vi "PH_SRDG645.calc Device Errors.vi"(1 "Device Errors out":cluster{"code":i32, "Text":string}[](array[cluster]), 2 "SRDG 645 error out":errorcluster) -> (0 "calculate Device Errors":cluster{"code":i32, "Text":string}[](array[cluster]))   [LabVIEW 2014, in "PH_SRDG645.lvlib"]
doc: "This VI calöculates the Device Errors; if \"Device Errors out\" are empty, \"SRDG 645 Error out\" is taken."
uses:
  PH_SRDG645.lvlib
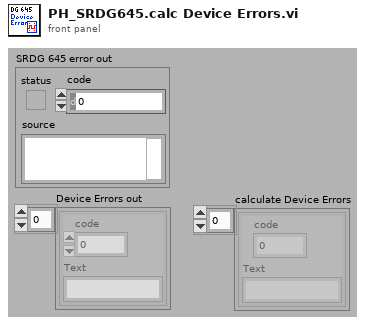
[diagram p1: front panel]
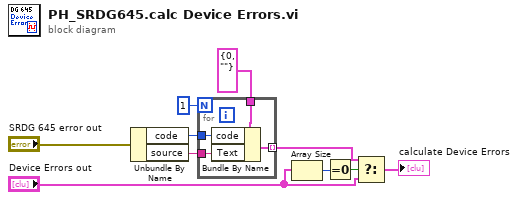
[diagram p0: block diagram]
diagram:
  n1 = Unbundle By Name("SRDG 645 error out") -> ("code"=w8:i32, "source"=w9:string)
  n2 = for {
    N: 1 -> [_]
    tunnel: [w14] -> w6 mode=indexing
    tunnel: cluster{"code":i32, "Text":string} {"code"=0, "Text"=""} ("Device Error") -> [w13]
    tunnel: w8 -> [w12]
    tunnel: w9 -> [w11]
    n3 = Bundle By Name(cluster=w13, "code"=w12, "Text"=w11) -> (w14:cluster{"code":i32, "Text":string})
  }
  n4 = Array Size(array="Device Errors out") -> (size(s)=w1:i32)
  n5 = Equal To 0?(x=w1) -> (x = 0?=w2:bool)
  n6 = Select(t=w6, s=w2, f="Device Errors out") -> (s? t:f=→"calculate Device Errors":cluster{"code":i32, "Text":string}[])
